vi "SVPO Limit Testing (N Ch) (SGL Waveform).vi"(7 "reset? (F)":bool, 9 "lower limit":sgl=-inf format="%.2f", 10 "upper limit":sgl=inf format="%.2f", 11 "signals in":waveform(sgl)[](array[waveform])) -> (1 "lower limit clearances":sgl[](array[numeric]) format="%.6f", 2 "upper limit clearances":sgl[](array[numeric]) format="%.6f", 3 "tests passed?":bool[](array[boolean]), 5 "timestamps":T1(array[cluster]))   [LabVIEW 2017, in "SoundVib_LimitTest.lvlib"]
doc: "Performs limit testing on single-precision waveforms, single-precision scaled arrays, or double-precision scalar measurements. You can specify an upper and lower boundary of the envelope to define a pass range. This VI uses the defined pass range to test the input signal. VI outputs apply to all the tests since the last VI reset. Use this VI on embedded targets that have limited computational resources. Wire data to the <B>value in</B> input to determine the polymorphic instance to use or manually select the instance."
uses:
  <vilib>/addons/Sound and Vibration/svt_Limit Test/SoundVib_LimitTest.lvlib
  <vilib>/addons/Sound and Vibration/svt_Limit Test/SVPO Limit Testing (1 Ch) (SGL Array) with IC.vi
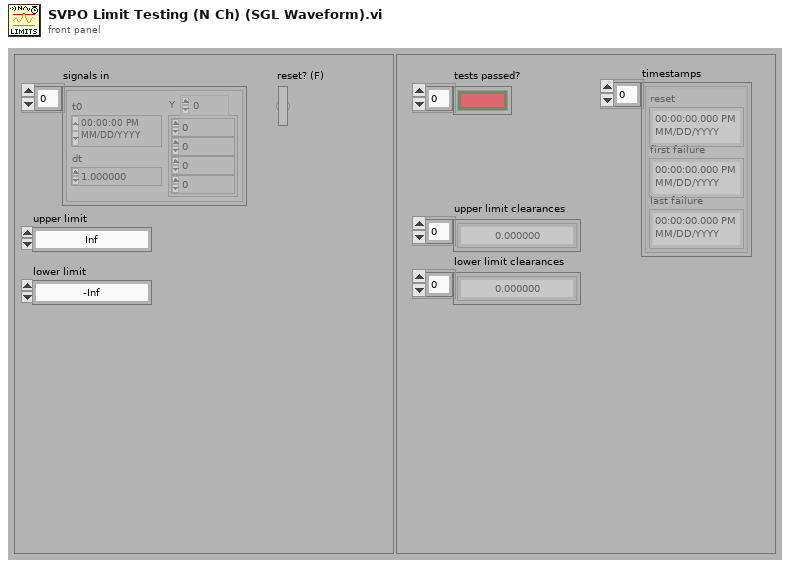
[diagram p1: front panel]
types:
  T1 = cluster{"reset":timestamp, "first failure":timestamp, "last failure":timestamp}[]
  T2 = typedef "svc_Waveform Limit State.ctl" = cluster{"timestamps":cluster{"reset":timestamp, "first failure":timestamp, "last failure":timestamp}, "limit state":T3}
  T3 = typedef "svc_SGL Limit State.ctl" = cluster{"upper limit clearance":sgl, "lower limit clearance":sgl, "test passed?":bool, "block passed?":bool}
  T4 = cluster{"reset":timestamp, "first failure":timestamp, "last failure":timestamp}
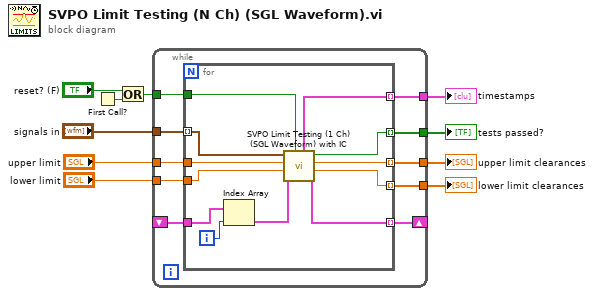
[diagram p0: block diagram]
diagram:
  n1 = First Call?() -> (First Call?: T/F=w6:bool)
  n2 = Or(x="reset? (F)", y=w6) -> (x .or. y?=w7:bool)
  n3 = while {
    tunnel: "signals in" -> [w21]
    tunnel: "upper limit" -> [w18]
    tunnel: "lower limit" -> [w17]
    tunnel: w7 -> [w20]
    shift-right: [w15] -> _
    shift-left: _ -> [w16]
    tunnel: [w14] -> w4
    tunnel: [w13] -> w3
    tunnel: [w12] -> w2
    tunnel: [w11] -> w1
    stop <- TRUE stop-if-true
    n4 = for {
      tunnel: w21 -> [w29] mode=indexing
      tunnel: w20 -> [w24]
      tunnel: w18 -> [w28]
      tunnel: w17 -> [w27]
      tunnel: w16 -> [w31]
      tunnel: [w32] -> w15 mode=indexing
      tunnel: [w26] -> w14 mode=indexing
      tunnel: [w25] -> w13 mode=indexing
      tunnel: [w23] -> w12 mode=indexing
      tunnel: [w22] -> w11 mode=indexing
      i -> [w33]
      n5 = Index Array(array=w31, index=w33) -> (element=w30:T2)
      n6 = call <vilib>:"SVPO Limit Testing (1 Ch) (SGL Waveform) with IC.vi"("reset? (F)"=w24, "initial conditions"=w30, "lower limit"=w27, "upper limit"=w28, "signal in"=w29) -> ("final conditions"=w32:T2, "lower limit clearance"=w25:sgl, "upper limit clearance"=w26:sgl, "test passed?"=w22:bool, "timestamps"=w23:T4)  [unwired: 2 in]
    }
  }
  "tests passed?" <- w1
  "upper limit clearances" <- w4
  "lower limit clearances" <- w3
  "timestamps" <- w2
